vi "Start OpenCLV.vi"(8 "Error In":errorcluster) -> (0 "Error Out":errorcluster)   [LabVIEW 2012]
doc: "Starts OpenCLV and clears any functional globals associated with OpenCLV, starts the error logging, and initializes the FFT library."
uses:
  OpenCLV x64.lvlib
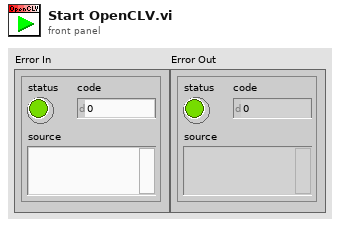
[diagram p1: front panel]
types:
  T1 = enum16{"Initialize", "Add Error", "View Error Log", "Save Error Log", "Set Verbose Mode", "Set Quite Mode"}
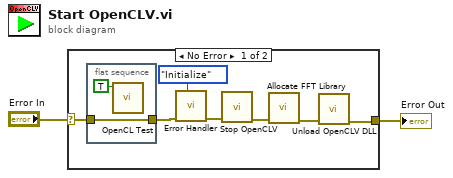
[diagram p0: block diagram]
diagram:
  n1 = case shown="No Error" "Error In" {
    selector: "Error In" -> [w4 w12]
    tunnel: [w7 w12] -> w1
    frame No Error {
      n2 = flat-sequence {
        tunnel: w4 -> [w10]
        tunnel: [w10] -> w3
        frame #0 {
          n3 = call "OpenCL Test.vi"("Init"=TRUE) -> ()  [unwired: 10 in, 1 out]
        }
      }
      n4 = call "Error Handler.vi"("Error Handler States"=T1."Initialize", "Error In"=w3) -> ("Error Out"=w6:errorcluster)  [unwired: 9 in]
      n5 = call "Stop OpenCLV.vi"("Error In"=w6) -> ("Error Out"=w9:errorcluster)  [unwired: 10 in]
      n6 = call "Allocate FFT Library.vi"("Error In"=w9) -> ("Error Out"=w8:errorcluster)  [unwired: 10 in]
      n7 = call "Unload OpenCLV DLL.vi"("Error In"=w8) -> ("Error Out"=w7:errorcluster)  [unwired: 10 in]
    }
    frame Error {
    }
  }
  "Error Out" <- w1
